vi "PH_AWG-510.contents.vi"   [LabVIEW 2014, in "PH_AWG-510.lvlib"]
uses:
  PH_AWG-510.lvlib
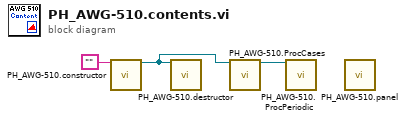
[diagram p0: block diagram]
diagram:
  n1 = call "PH_AWG-510.constructor.vi"("name"="") -> ("i ref out"=w1:refnum<vi>)  [unwired: 16 in, 2 out]
  n2 = call "PH_AWG-510.destructor.vi"("i ref in"=w1) -> ()  [unwired: 18 in, 1 out]
  n3 = call "PH_AWG-510.ProcCases.vi"("i ref in"=w1) -> ("i ref out"=w3:refnum<vi>)  [unwired: 16 in, 2 out]
  n4 = call "PH_AWG-510.ProcPeriodic.vi"("i ref in"=w3) -> ()  [unwired: 16 in, 3 out]
  n5 = call "PH_AWG-510.panel.vi"() -> ()  [unwired: 19 in, 1 out]
